vi "Send Programmatic Value Change.vi"(6 "Datum Name":string, 8 "error in (no error)":errorcluster, 9 "New Value":variant, 10 "Event Time (Auto)":u32, 11 "Message Enqueuer in":refnum<class "Message Enqueuer.lvclass">) -> (0 "error out":errorcluster)   [LabVIEW 2015, in "ActorAutoRegistration.lvlib" / "ValueChangeMsg.lvclass"]
doc: "<License>\nCopyright © 2017 Composed Systems, LLC | All rights reserved\nwww.composed.io\n\nAuthor: Ethan Stern <ethan.stern@composed.io>\n\nThis software is provided \"AS IS\" WITHOUT WARRANTIES, either express or implied, AND IS FOR EDUCATIONAL PURPOSES ONLY.\n</License>"
uses:
  ValueChangeMsg.lvclass
  <vilib>/ActorFramework/Message Enqueuer/Message Enqueuer.lvclass
  ValueChangeMsg.lvclass/ValueChangeMsg.ctl
  EventDataMessage/EventDataMessage.lvclass
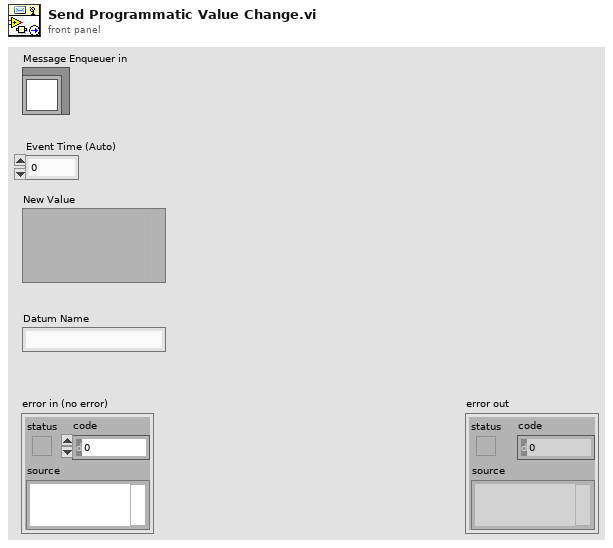
[diagram p1: front panel]
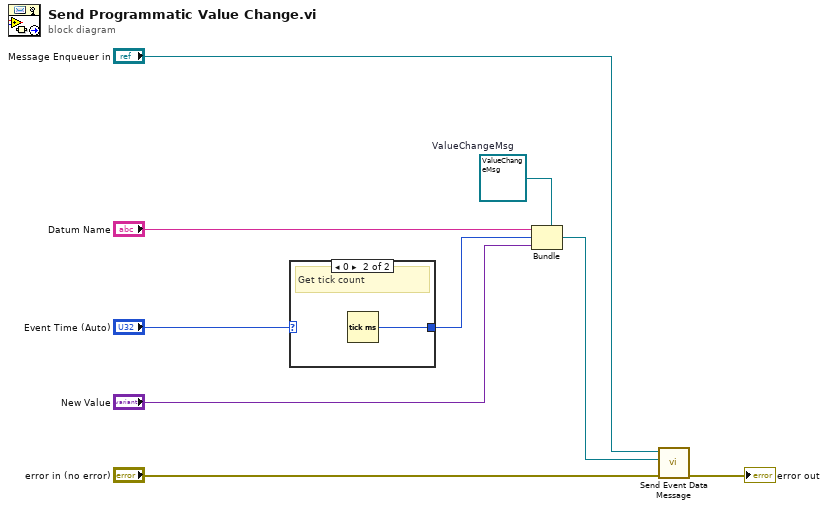
[diagram p0: block diagram]
diagram:
  w9 = refnum<class "ValueChangeMsg.lvclass"> refnum  # ValueChangeMsg
  n1 = case shown="0" "Event Time (Auto)" {
    selector: "Event Time (Auto)" -> [w10 _]
    tunnel: [w10 w11] -> w3
    frame 1.. {
      # "Time input was wired"
    }
    frame 0 {
      # "Get tick count"
      n2 = Tick Count (ms)() -> (millisecond timer value=w11:u32)
    }
  }
  n3 = Bundle(cluster=w9, "Datum Name", w3, "New Value") -> (w6:refnum<class "ValueChangeMsg.lvclass">)
  n4 = call "Send Event Data Message.vi"("error in (no error)"="error in (no error)", "EventDataMessage in"=w6, "Message Enqueuer in"="Message Enqueuer in") -> ("error out"=→"error out":errorcluster)  [unwired: 8 in]
